vi "fetch_and_translate_trigger.vi"(8 "error in (no error)":errorcluster, 11 "ImageAssemblerDL090211Scaffold in":refnum<class "ImageAssemblerDL090211Scaffold.lvclass">) -> (0 "error out":errorcluster, 1 "sender TLC type":T1, 2 "internal trigger":T2, 3 "ImageAssemblerDL090211Scaffold out":refnum<class "ImageAssemblerDL090211Scaffold.lvclass">)   [LabVIEW 2010, in "ImageAssemblerDL090211Scaffold.lvclass"]
uses:
  ImageAssemblerDL090211Scaffold.lvclass
  action_enum.ctl
  common/enumerations/top-level_component_type_enum.ctl
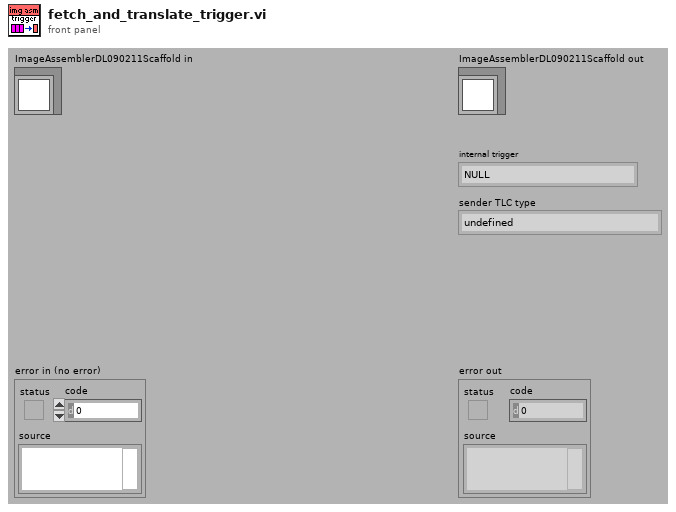
[diagram p1: front panel]
types:
  T1 = typedef "top-level_component_type_enum.ctl" = enum16{"undefined", "ImagingMode", "ScanHead", "DAQ", "ImageAssembler", "Display", "DataCollection", "Analyser", "Stimulator", "ExperimentController", "Instrument", "Stage"}
  T2 = typedef "ImageAssemblerDL090211Scaffold.lvclass/action_enum.ctl" = enum16{"NULL", "initialise", "terminate", "start", "stop", "insert", "send", "attach observer", "register as observer", "detach observer"}
  T3 = typedef "GenericToplevelComponent.lvclass/common_trigger_enum.ctl" = enum16{"NULL", "initialise", "terminate", "fetch command", "fetch data", "attach observer", "register as observer", "detach observer", "acknowledge", "start", "stop", "sweep started", "sweep finished", "experiment started", "experiment stopped"}
  T4 = typedef "trigger_type_enum.ctl" = enum8{"external", "internal", "common"}
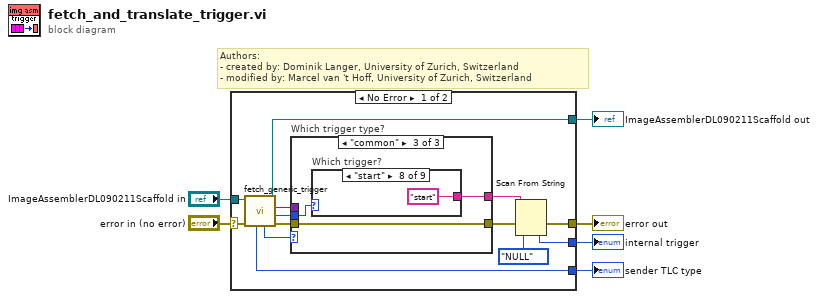
[diagram p0: block diagram]
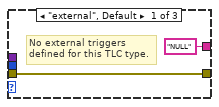
[diagram p2: hidden frame]
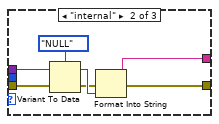
[diagram p3: hidden frame]
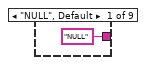
[diagram p4: hidden frame]
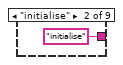
[diagram p5: hidden frame]
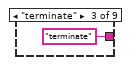
[diagram p6: hidden frame]
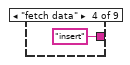
[diagram p7: hidden frame]
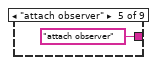
[diagram p8: hidden frame]
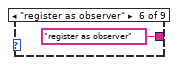
[diagram p9: hidden frame]
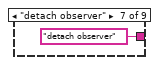
[diagram p10: hidden frame]
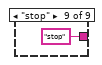
[diagram p11: hidden frame]
diagram:
  # "Authors: \n- created by: Dominik Langer, University of Zurich, Switzerland\n- modified by: Marcel van 't Hoff, University of Zurich, Switzerland"
  n1 = case shown="No Error" "error in (no error)" {
    selector: "error in (no error)" -> [w19 w42]
    tunnel: [w10 w42] -> w5
    tunnel: [w15 w41] -> w3
    tunnel: "ImageAssemblerDL090211Scaffold in" -> [w16 w41]
    tunnel: [w7 _] -> w2
    tunnel: [w12 _] -> w1
    frame No Error {
      n2 = call-dynamic "fetch_generic_trigger.vi"("error in (no error)"=w19, "GenericToplevelComponent in"=w16) -> ("error out"=w18:errorcluster, "common trigger"=w13:T3, "trigger"=w14:variant, "GenericToplevelComponent out"=w15:refnum<class "ImageAssemblerDL090211Scaffold.lvclass">, "trigger type"=w17:T4, "sender TLC type"=w12:T1)  [unwired: 3 in, 1 out]
      n3 = case "Which trigger type?" shown="\"common\"" w17 {
        tunnel: w18 -> [w21 w27 w31]
        tunnel: [w21 w22 w31] -> w9
        tunnel: w14 -> [_ w28 _]
        tunnel: w13 -> [_ _ w30]
        tunnel: ["NULL" w24 w29] -> w11
        frame "external", Default {
          # "No external triggers defined for this TLC type."
        }
        frame "internal" {
          n4 = Variant To Data(error in=w27, Variant=w28, type=action_enum."NULL") -> (error out=w23:errorcluster, data=w25:T2)
          n5 = Format Into String(error in=w23, w25) -> (resulting string=w24:string, error out=w22:errorcluster)  [unwired: 2 in]
        }
        frame "common" {
          n6 = case "Which trigger?" shown="\"start\"" w30 {
            tunnel: ["NULL" "initialise" "terminate" "insert" "attach observer" "register as observer" "detach observer" "start" "stop"] -> w29
            frame "NULL", Default {
            }
            frame "initialise" {
            }
            frame "terminate" {
            }
            frame "fetch data" {
            }
            frame "attach observer" {
            }
            frame "register as observer" {
            }
            frame "detach observer" {
            }
            frame "start" {
            }
            frame "stop" {
            }
          }
        }
      }
      n7 = Scan From String(input string=w11, error in=w9, default 1=action_enum."NULL" ("internal trigger")) -> (error out=w10:errorcluster, output 1=w7:T2)  [unwired: 2 in, 2 out]
    }
    frame Error {
    }
  }
  "error out" <- w5
  "ImageAssemblerDL090211Scaffold out" <- w3
  "internal trigger" <- w2
  "sender TLC type" <- w1
